vi "18.vi"() -> ()   [LabVIEW 2012]
uses:
  <vilib>/addons/control/pid/pid.llb/PID (DBL).vi
  <vilib>/express/express arith-compare/Formula/XNode/ExpressFormulaBlockNode.xnode
  <vilib>/addons/control/pid/NI_PID_pid.lvlib
panel:
  in  "k2":dbl
  in  "c2":dbl
  in  "m2":dbl
  in  "c1":dbl
  in  "m1":dbl
  in  "k1":dbl
  out "z2":dbl
  out "z2_dot":dbl
  out "(z1-z2)dot":dbl
  out "z1-z2":dbl
  out "z1_dot":dbl
  out "z1":dbl
  in  "disturbance input(w)":dbl
  in  "control input(u)":dbl
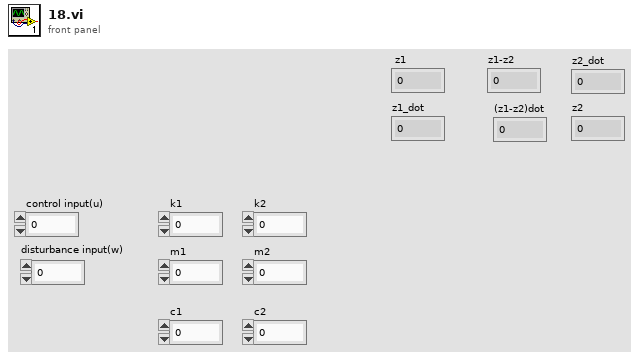
[diagram p1: front panel]
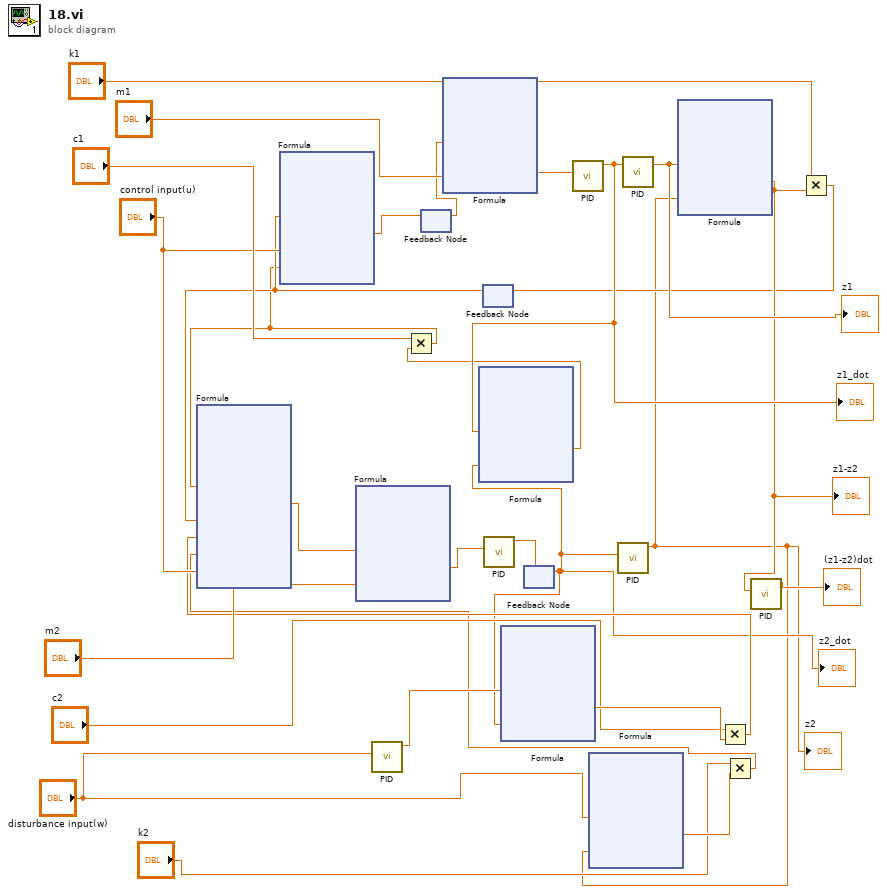
[diagram p0: block diagram]
diagram:
  n1 = call-poly <vilib>:"PID.vi"("process variable"="disturbance input(w)") -> ("output"=w20:dbl)  [unwired: 9 in, 1 out]
  n2 = feedback #1() -> (w24:dbl)  [unwired: 1 in]
  n3 = xnode "Formula"("X1"=w24, "X2"="m1") -> ("Result"=w29:dbl)  [unwired: 1 in, 1 out]
  n4 = feedback #2() -> (w6:dbl)  [unwired: 1 in]
  n5 = feedback #3() -> (w3:dbl)  [unwired: 1 in]
  "z2_dot" <- w3
  n6 = xnode "Formula"("X1"=w20, "X2"=w3) -> ("Result"=w15:dbl)  [unwired: 1 in, 1 out]
  n7 = call-poly <vilib>:"PID.vi"("process variable"=w29) -> ("output"=w22:dbl)  [unwired: 9 in, 1 out]
  "z1_dot" <- w22
  n8 = xnode "Formula"("X1"=w22, "X2"=w3) -> ("Result"=w21:dbl)  [unwired: 1 in, 1 out]
  n9 = Multiply(x="c1", y=w21) -> (x*y=w5:dbl)
  n10 = xnode "Formula"("X1"=w6, "X2"="control input(u)", "X3"=w5) -> ("Result"=w25:dbl)  [unwired: 1 in, 1 out]
  n11 = feedback-in #1(w25) -> ()
  n12 = call-poly <vilib>:"PID.vi"("process variable"=w3) -> ("output"=w1:dbl)  [unwired: 9 in, 1 out]
  "z2" <- w1
  n13 = xnode "Formula"("X1"="disturbance input(w)", "X2"=w1) -> ("Result"=w12:dbl)  [unwired: 1 in, 1 out]
  n14 = call-poly <vilib>:"PID.vi"("process variable"=w22) -> ("output"=w27:dbl)  [unwired: 9 in, 1 out]
  "z1" <- w27
  n15 = xnode "Formula"("X1"=w27, "X2"=w1) -> ("Result"=w9:dbl)  [unwired: 1 in, 1 out]
  "z1-z2" <- w9
  n16 = Multiply(x="c2", y=w15) -> (x*y=w13:dbl)
  n17 = Multiply(x="k2", y=w12) -> (x*y=w10:dbl)
  n18 = xnode "Formula"("X1"=w5, "X2"=w6, "X3"=w13, "X4"=w10, "X5"="control input(u)") -> ("Result"=w17:dbl)  [unwired: 1 in, 1 out]
  n19 = xnode "Formula"("X1"=w17, "X2"="m2") -> ("Result"=w19:dbl)  [unwired: 1 in, 1 out]
  n20 = call-poly <vilib>:"PID.vi"("process variable"=w19) -> ("output"=w4:dbl)  [unwired: 9 in, 1 out]
  n21 = feedback-in #3(w4) -> ()
  n22 = call-poly <vilib>:"PID.vi"("process variable"=w9) -> ("output"=→"(z1-z2)dot":dbl)  [unwired: 9 in, 1 out]
  n23 = Multiply(x="k1", y=w9) -> (x*y=w7:dbl)
  n24 = feedback-in #2(w7) -> ()
